vi "CSM Class API Arguments Type in Short.vi"(11 "String":string) -> (3 "s? t:f":string)   [LabVIEW 2020, in "CSM Mermaid Support.lvlib"]
uses:
  CSM Mermaid Support.lvlib
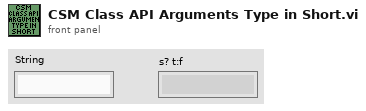
[diagram p1: front panel]
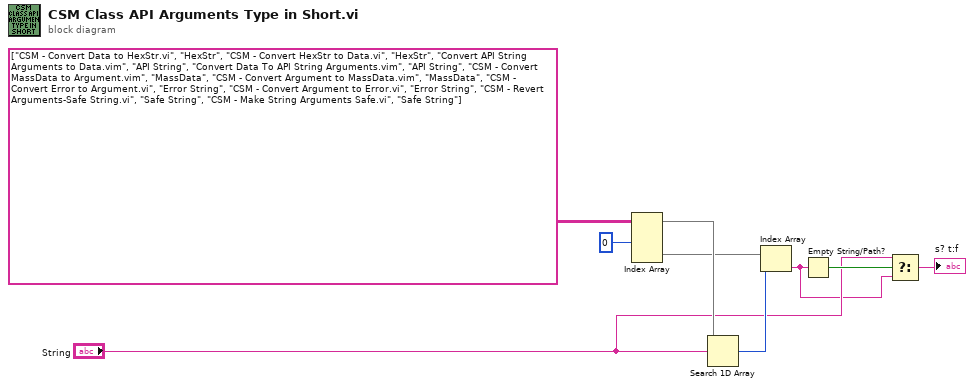
[diagram p0: block diagram]
diagram:
  n1 = Index Array(array=string[][] [["CSM - Convert Data to HexStr.vi", "HexStr"], ["CSM - Convert HexStr to Data.vi", "HexStr"], ["Convert API String Arguments to Data.vim", "API String"], ["Convert Data To API String Arguments.vim", "API String"], ["CSM - Convert MassData to Argument.vim", "MassData"], ["CSM - Convert Argument to MassData.vim", "MassData"], ["CSM - Convert Error to Argument.vi", "Error String"], ["CSM - Convert Argument to Error.vi", "Error String"], ["CSM - Revert Arguments-Safe String.vi", "Safe String"], ["CSM - Make String Arguments Safe.vi", "Safe String"]], index (col) #1=0 ("disabled index (col)")) -> (element #1=w8:string[], element #2=w5:string[])  [unwired: 3 in]
  n2 = Search 1D Array(1D array=w8, element="String") -> (index of element=w6:i32)  [unwired: 1 in]
  n3 = Index Array(array=w5, index=w6) -> (element=w2:string)
  n4 = Empty String/Path?(string/path=w2) -> (empty?=w4:bool)
  n5 = Select(t="String", s=w4, f=w2) -> (s? t:f=→"s? t:f":string)
